vi "Interface.vi"(9 "EventsIn":T1, 10 "Events":T2) -> ()   [LabVIEW 2014, in "VIWindowProperties.lvlib" / "VIWindowProperties.lvclass"]
uses:
  VIWindowProperties.lvclass
  Framework/_Plugins/_LVCMPlugin/GCMPlugin_EventsOut.ctl
  Framework/_Plugins/_LVCMPlugin/GCMPlugin_EventsIn.ctl
  <vilib>/Utility/miscctls.llb/LVPointTypeDef.ctl
  Framework/_Plugins/GCMPlugin/GCMPlugin.lvclass
panel:
  in  "ToAP":bool
  in  "ToSP":bool
  in  "Tab Control":enum32{"Appearance", "Size and Position"}(tab)
  in  "Window has title bar":bool
  in  "Window behavior":enum32{"Default", "Floating", "Modal"}(radio)
  in  "Hide when LabVIEW in not active":bool
  in  "Window runs transparently":bool
  in  "Show menu bar":bool
  in  "Show vertical scroll bar":bool
  in  "Show horizontal scroll bar":bool
  in  "Show toolbar when running":bool
  in  "Show Abort button":bool
  in  "Show Run button":bool
  in  "Show Run Continuously":bool
  in  "Show front panel when called":bool
  in  "Close afterwards if originally closed":bool
  in  "Show front panel when loaded":bool
  in  "Transparently":u8 caption="Numeric Control"
  in  "Allow user to close window":bool
  in  "Allow user to resize window":bool
  in  "Allow user to minimalize window":bool
  in  "Allow default run time shortcut menus":bool
  in  "Highlight Enter boolean":bool
  in  "SP_SetCurrentSize":bool
  in  "SP_Height":i16 caption="Height"
  in  "SP_Width":i16 caption="Width"
  in  "SP_UseCurSize":bool caption="Use Current Panel Size"
  in  "SP_SetCurrentPos":bool
  in  "SP_Left":i16 caption="Left"
  in  "SP_Top":i16 caption="Top"
  in  "SP_UseCurPos":bool caption="Use Current Position"
  in  "SP_Scale":bool caption="Scale all objects on front panel as the window resizes"
  in  "SP_MinHeight":i16 caption="Height"
  in  "SP_MinWidth":i16 caption="Width"
  in  "SP_SetMinCurrent":bool
  in  "SP_proportions":bool caption="Maintain proportions of window for different monitor resolutions"
  in  "SP_Position":u16(ring) caption="Position" items=["Unchanged", "Centered", "Maximized", "Minimized", "Custom"]
  in  "SP_Monitor":u16(ring) caption="Monitor" items=["Primary", "1", "2", "3"]
  # "Window Size"
  # "Minimum Panel Size"
  # "Window Run-Time Position"
  # "Window Position"
  # "Panel Size"
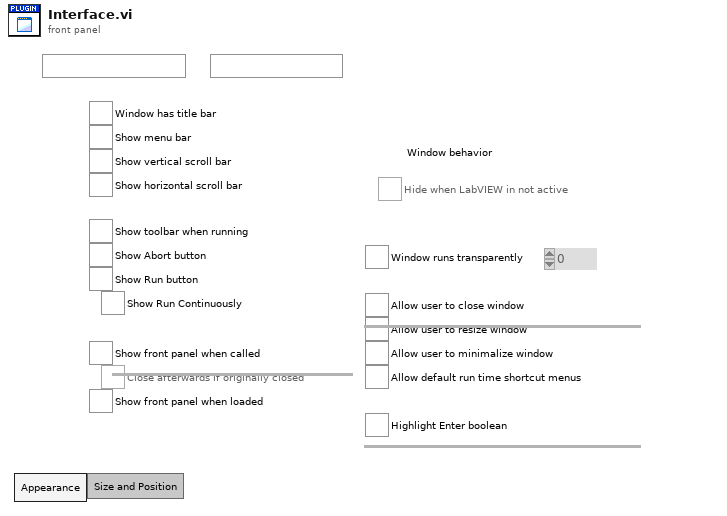
[diagram p1: front panel]
types:
  T1 = typedef "GCMPlugin.lvclass/GCMPlugin_EventsIn.ctl" = cluster{"Stop":refnum<user-event>, "ItemSelected":refnum<user-event>, "ItemDeselected":refnum<user-event>, "PluginActivated":refnum<user-event>, "PluginDeactivated":refnum<user-event>}
  T2 = typedef "GCMPlugin.lvclass/GCMPlugin_EventsOut.ctl" = cluster{"ItemEdited":refnum<user-event>}
  T3 = enum16{"No Scaling", "Scale All Objects", "Scale Single Object"}
  T4 = enum8{"Enabled", "Disabled", "Disabled and Grayed Out"}
  T5 = enum16{"Always On", "Always Off", "Off While Running"}
  T6 = typedef "LVPointTypeDef.ctl" = cluster{"Horizontal":i16, "Vertical":i16}
  T7 = enum32{"Invalid", "Default", "Floating", "Floating/Auto-Hide", "Modal"}
  T8 = enum32{"Unchanged", "Centered", "Maximized", "Minimized", "Custom"}
  T9 = typedef "LVRectTypeDef.ctl" = cluster{"Left":i16, "Top":i16, "Right":i16, "Bottom":i16}
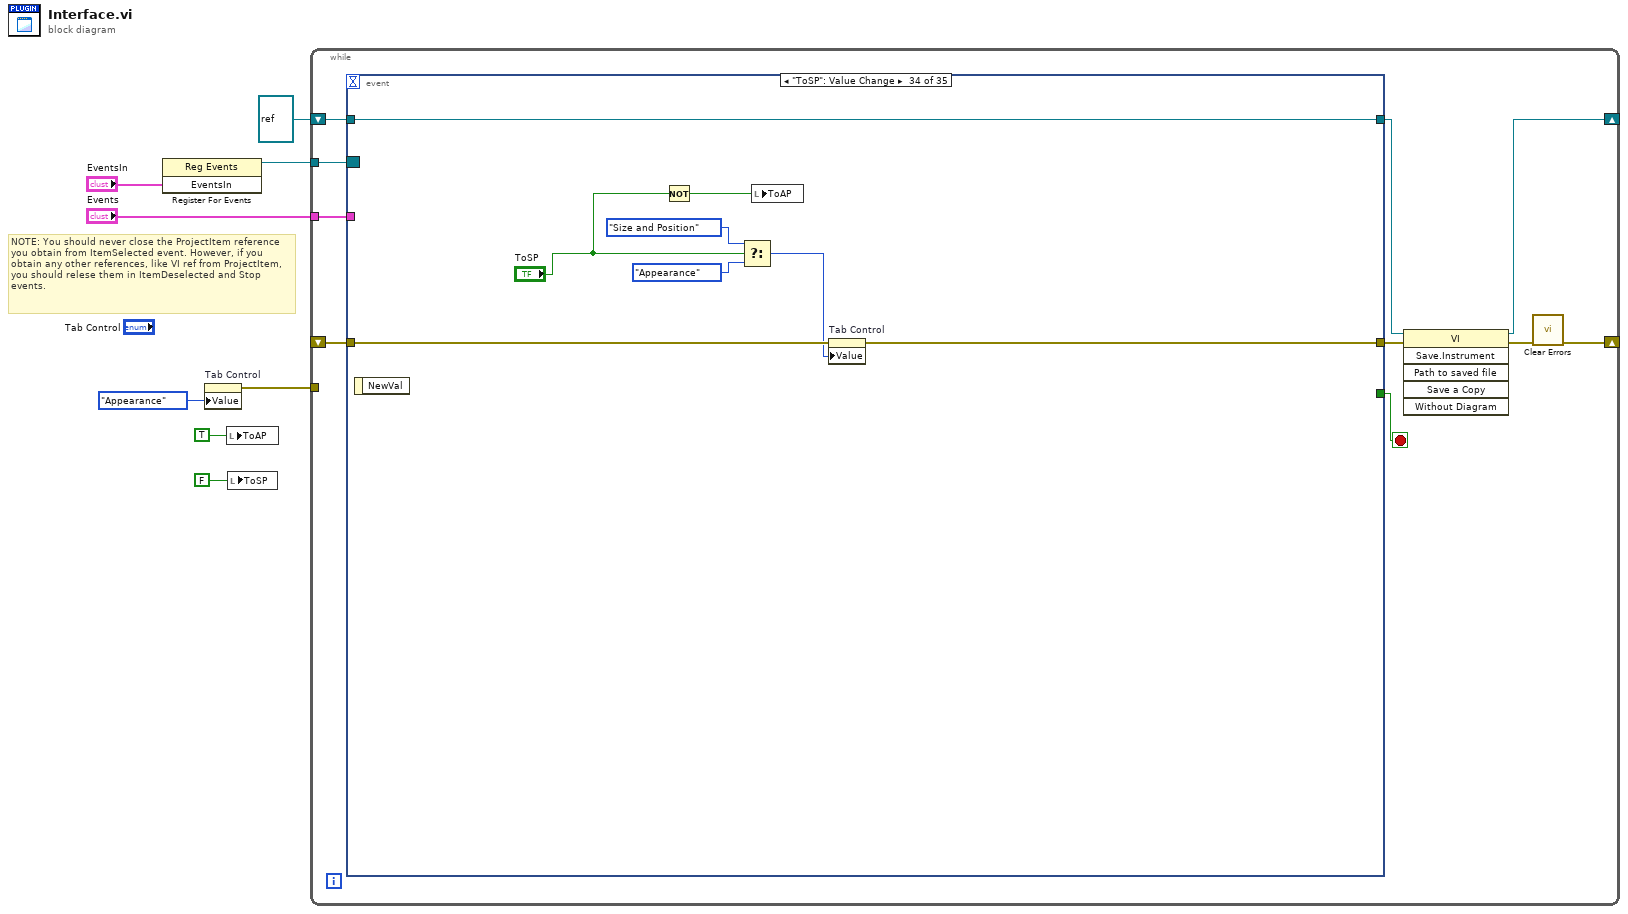
[diagram p0: block diagram]
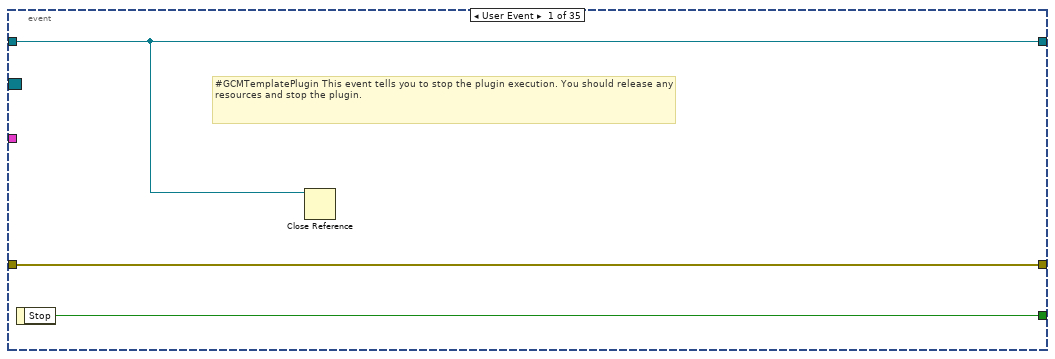
[diagram p2: hidden frame]
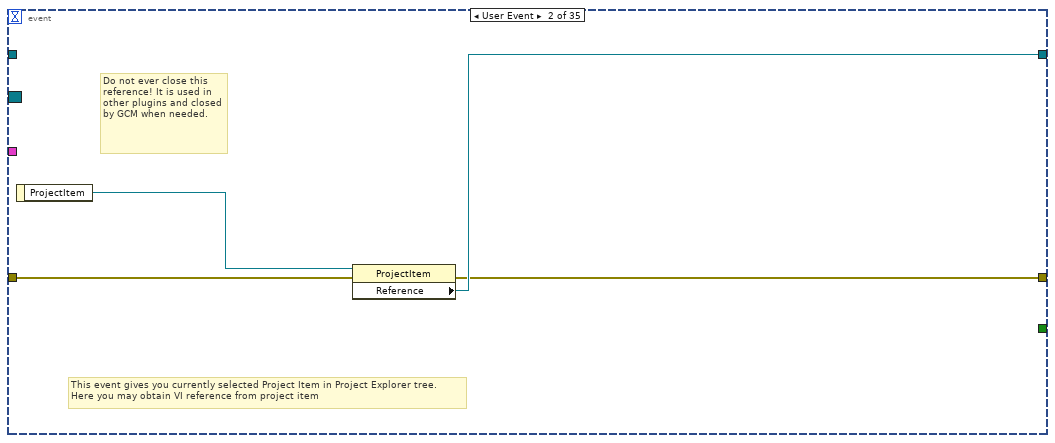
[diagram p3: hidden frame]
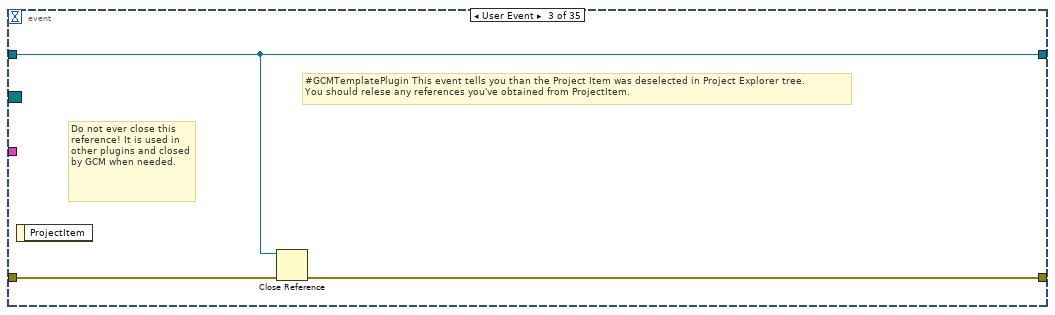
[diagram p4: hidden frame]
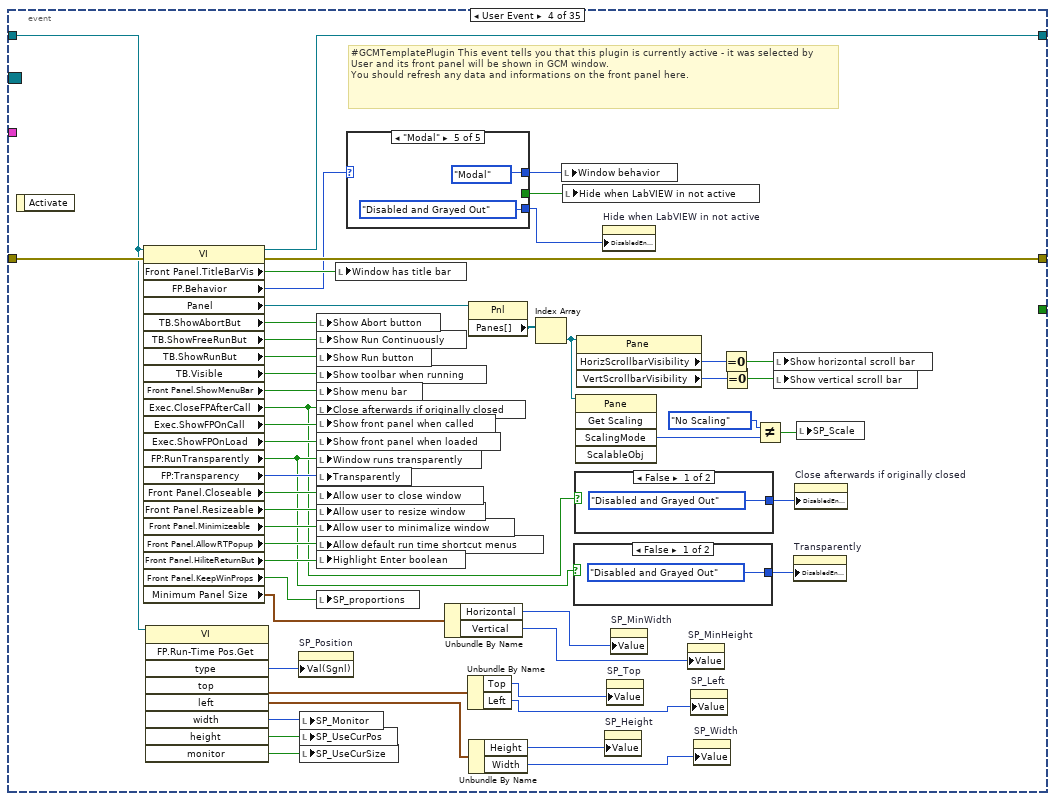
[diagram p5: hidden frame]
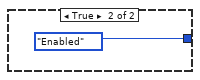
[diagram p6: hidden frame]
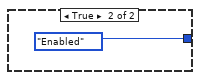
[diagram p7: hidden frame]
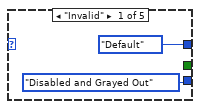
[diagram p8: hidden frame]
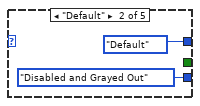
[diagram p9: hidden frame]
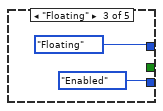
[diagram p10: hidden frame]
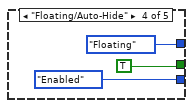
[diagram p11: hidden frame]
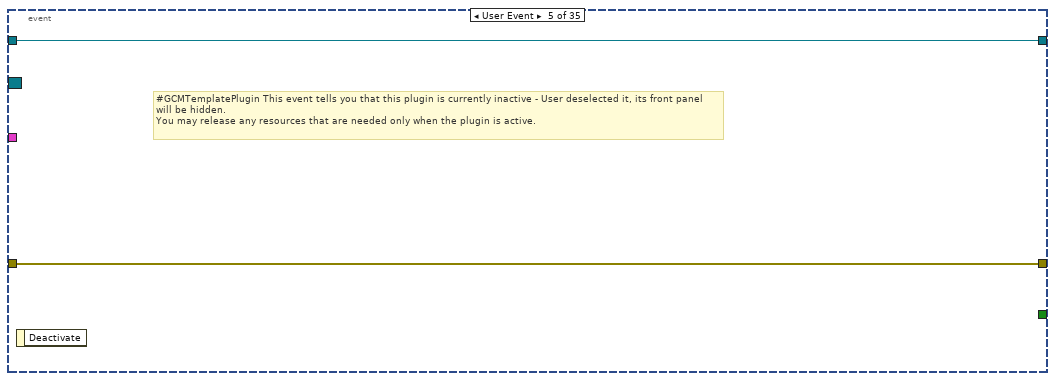
[diagram p12: hidden frame]
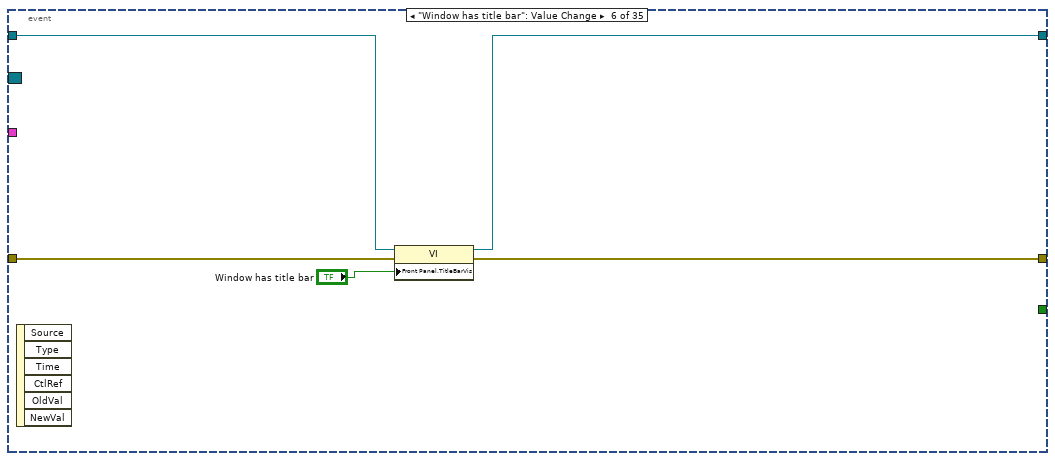
[diagram p13: hidden frame]
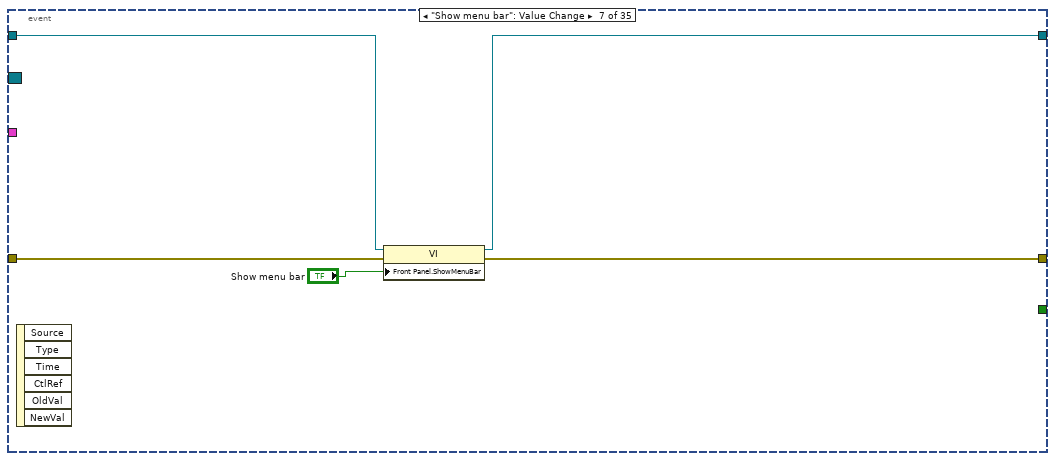
[diagram p14: hidden frame]
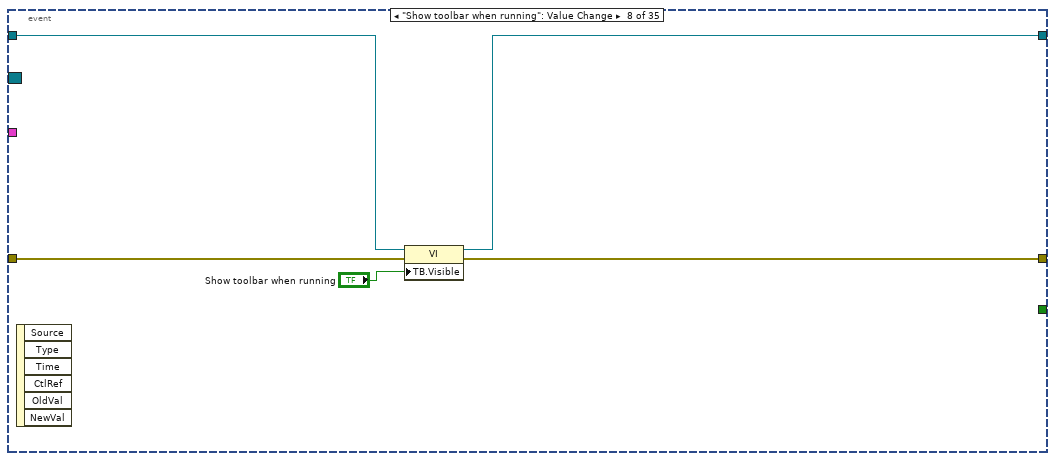
[diagram p15: hidden frame]
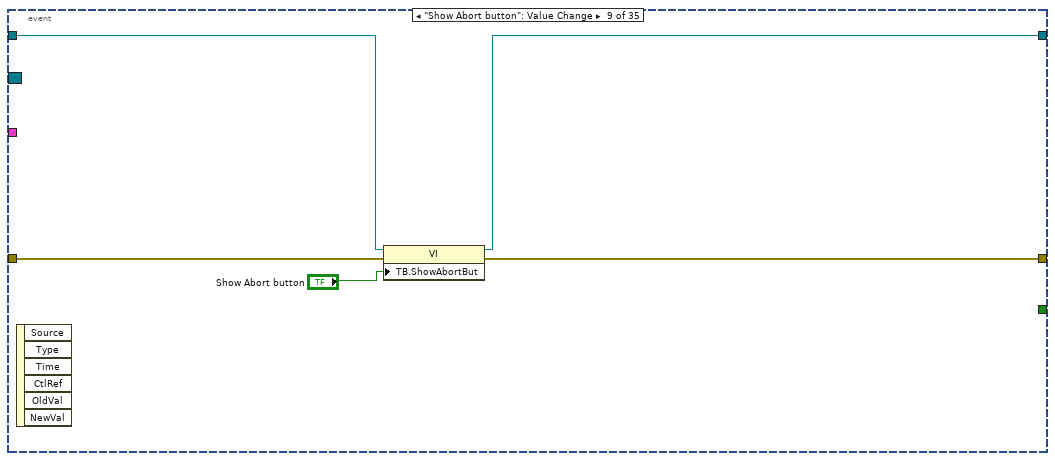
[diagram p16: hidden frame]
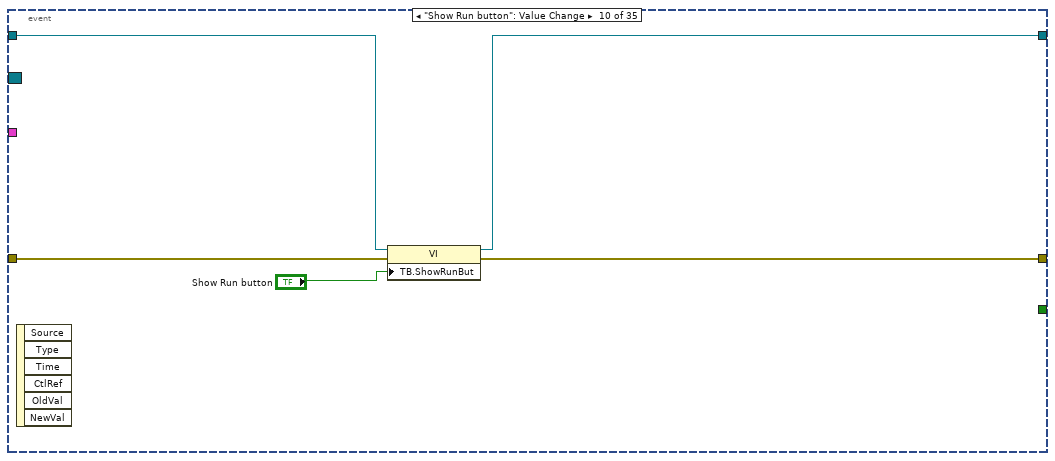
[diagram p17: hidden frame]
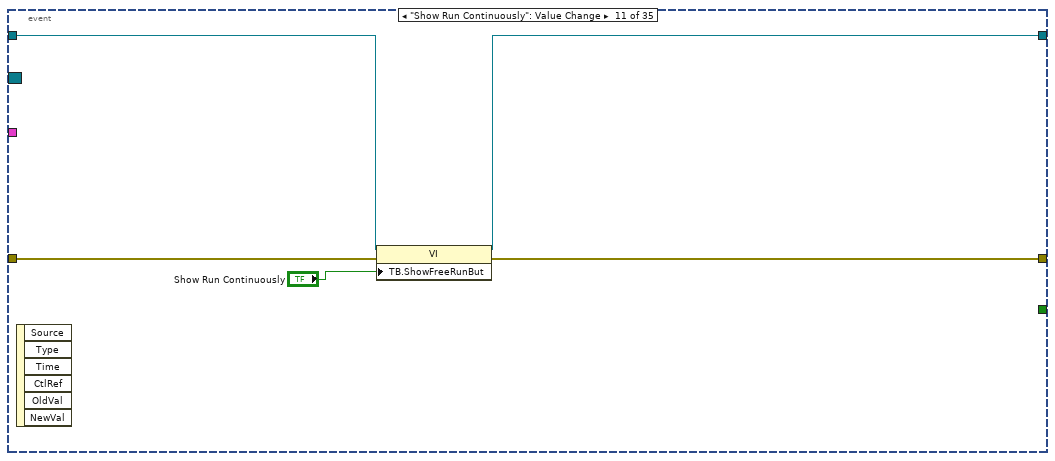
[diagram p18: hidden frame]
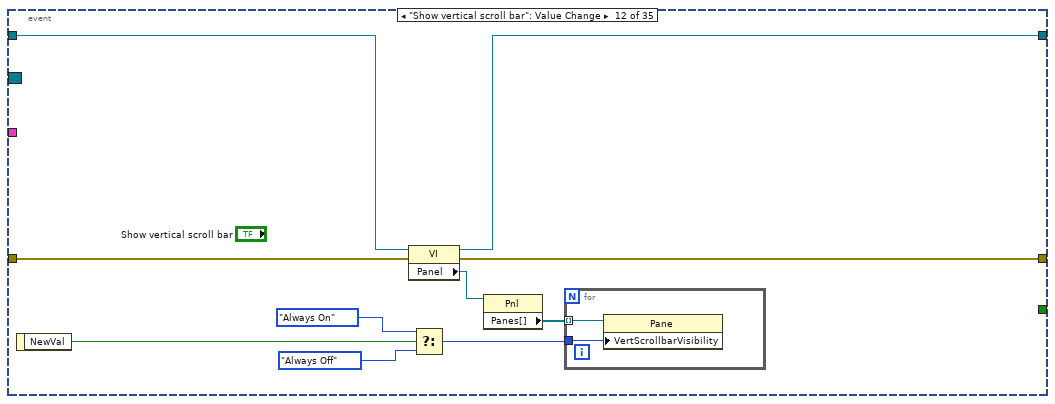
[diagram p19: hidden frame]
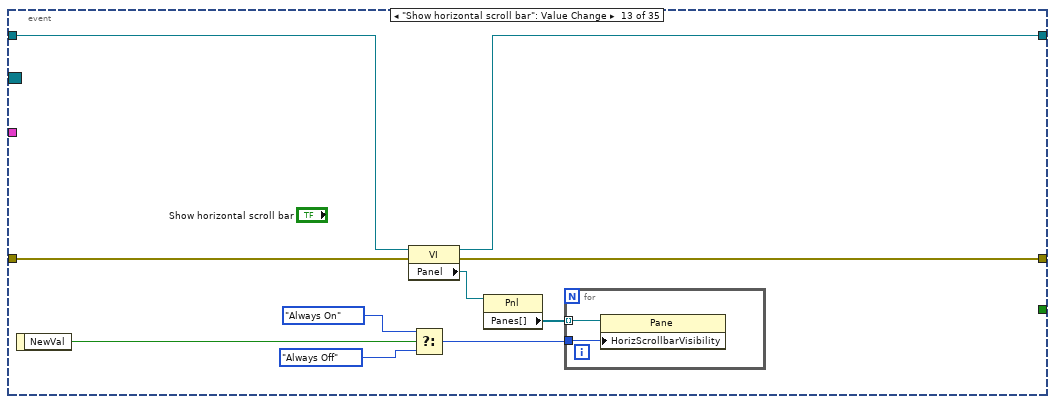
[diagram p20: hidden frame]
diagram:
  # "NOTE: You should never close the ProjectItem reference you obtain from ItemSelected event. However, if you obtain any other references, like VI ref from ProjectItem, you should relese them in ItemDeselected and Stop events."
  n1 = register-events("EventsIn") -> (reference out=w7:refnum<event-registration>)  [unwired: 2 in, 1 out]
  n2 = property on="Tab Control" class="TabCtl (strict)"("Value"=enum32{"Appearance", "Size and Position"}."Appearance" ("Tab Control")) -> (error out=w3:errorcluster)  [unwired: 2 in, 1 out]
  n3 = local write "ToAP"(TRUE ("ToAP")) -> ()
  n4 = local write "ToSP"(FALSE ("ToAP")) -> ()
  n5 = while {
    tunnel: w7 -> [w18]
    tunnel: "Events" -> [w17]
    shift-right: [w9] -> _
    shift-left: refnum<vi> refnum ("Reference") -> [w15]
    shift-right: [w12] -> _
    shift-left: _ -> [w13]
    tunnel: w3 -> [_]
    stop <- w16 stop-if-true
    n6 = event shown="[33] \"ToSP\": Value Change" {
      selector: w18 -> [_ _ _ _ _ _ _ _ _ _ _ _ _ _ _ _ _ _ _ _ _ _ _ _ _ _ _ _ _ _ _ _ _ _ _]
      dyn-events: _ -> [_ _ _ _ _ _ _ _ _ _ _ _ _ _ _ _ _ _ _ _ _ _ _ _ _ _ _ _ _ _ _ _ _ _ _]
      timeout: _ -> [_ _ _ _ _ _ _ _ _ _ _ _ _ _ _ _ _ _ _ _ _ _ _ _ _ _ _ _ _ _ _ _ _ _ _]
      tunnel: w17 -> [_ _ _ _ _ _ _ _ _ _ _ _ _ _ _ _ _ _ _ _ _ _ _ _ _ _ _ _ _ _ _ _ _ _ _]
      tunnel: [w21 _ _ _ _ _ _ _ _ _ _ _ _ _ _ _ _ _ _ _ _ _ _ _ _ _ _ _ _ _ _ _ _ _ _] -> w16
      tunnel: [w19 w24 w28 w75 w95 w97 w102 w107 w112 w117 w122 w132 w144 w153 w160 w165 w172 w179 w184 w189 w194 w199 w204 w209 w217 w234 w350 w355 w376 w399 w406 w417 w423 w443 w451] -> w10
      tunnel: w15 -> [w19 _ w28 w39 w95 w98 w103 w108 w113 w118 w123 w133 w145 w154 w161 w166 w173 w180 w185 w190 w195 w200 w205 w210 w218 w235 w347 w354 w375 w398 w405 w408 w424 w443 w451]
      tunnel: [w20 w23 w26 w77 w94 w99 w104 w109 w114 w119 w124 w134 w146 w155 w162 w167 w174 w181 w186 w191 w196 w201 w206 w211 w219 w236 w351 w356 w377 w400 w407 w416 w425 w441 w449] -> w14
      tunnel: w13 -> [w20 w22 w27 w78 w94 w100 w105 w110 w115 w120 w125 w135 w147 w156 w163 w168 w175 w182 w187 w192 w197 w202 w207 w212 w220 w237 w346 w353 w374 w397 w404 w418 w426 w442 w450]
      event User Event {
        # "#GCMTemplatePlugin This event tells you to stop the plugin execution. You should release any resources and stop the plugin."
        n7 = event-data() -> ("Stop"=w21:bool)  [unwired: 1 in]
        n8 = Close Reference(reference=w19) -> ()  [unwired: 1 in, 1 out]
      }
      event User Event {
        # "Do not ever close this reference! It is used in other plugins and closed by GCM when needed."
        # "This event gives you currently selected Project Item in Project Explorer tree.\nHere you may obtain VI reference from project item"
        n9 = event-data() -> ("ProjectItem"=w25:refnum<vi>)  [unwired: 1 in]
        n10 = property class="ProjectItem"(reference=w25, error in=w22) -> (error out=w23:errorcluster, "Reference"=w24:refnum<vi>)  [unwired: 1 out]
      }
      event User Event {
        # "Do not ever close this reference! It is used in other plugins and closed by GCM when needed."
        # "#GCMTemplatePlugin This event tells you than the Project Item was deselected in Project Explorer tree.\nYou should relese any references you've obtained from ProjectItem."
        n11 = event-data() -> ()  [unwired: 1 in, 1 out]
        n12 = Close Reference(reference=w28, error in (no error)=w27) -> (error out=w26:errorcluster)
      }
      event User Event {
        # "#GCMTemplatePlugin This event tells you that this plugin is currently active - it was selected by User and its front panel will be shown in GCM window.\nYou should refresh any data and informations on the front panel here."
        n13 = event-data() -> ()  [unwired: 1 in, 1 out]
        n14 = property class="VI"(reference=w39, error in=w78) -> (reference out=w75:refnum<vi>, error out=w77:errorcluster, "Front Panel.TitleBarVis"=w76:bool, "FP.Behavior"=w54:T7, "Panel"=w60:refnum<vi>, "TB.ShowAbortBut"=w70:bool, "TB.ShowFreeRunBut"=w71:bool, "TB.ShowRunBut"=w72:bool, "TB.Visible"=w73:bool, "Front Panel.ShowMenuBar"=w69:bool, "Exec.CloseFPAfterCall"=w49:bool, "Exec.ShowFPOnCall"=w68:bool, "Exec.ShowFPOnLoad"=w67:bool, "FP:RunTransparently"=w51:bool, "FP:Transparency"=w66:u8, "Front Panel.Closeable"=w65:bool, "Front Panel.Resizeable"=w64:bool, "Front Panel.Minimizeable"=w63:bool, "Front Panel.AllowRTPopup"=w62:bool, "Front Panel.HiliteReturnBut"=w61:bool, "Front Panel.KeepWinProps"=w47:bool, "Minimum Panel Size"=w42:T6)
        n15 = invoke class="VI" method="FP.Run-Time Pos.Get"(reference=w39) -> ("type"=w35:T8, "top"=w34:cluster{"Top":i16, "Left":i16}, "left"=w31:cluster{"Height":i16, "Width":i16}, "width"=w38:i16, "height"=w37:bool, "monitor"=w36:bool)  [unwired: 8 in, 3 out]
        n16 = property on="SP_Position" class="Ring (strict)"("Val(Sgnl)"=w35) -> ()  [unwired: 2 in, 2 out]
        n17 = local write "SP_Monitor"(w38) -> ()
        n18 = local write "SP_UseCurPos"(w37) -> ()
        n19 = local write "SP_UseCurSize"(w36) -> ()
        n20 = local write "Show Abort button"(w70) -> ()
        n21 = local write "Show Run Continuously"(w71) -> ()
        n22 = local write "Show Run button"(w72) -> ()
        n23 = local write "Show toolbar when running"(w73) -> ()
        n24 = local write "Show menu bar"(w69) -> ()
        n25 = local write "Close afterwards if originally closed"(w49) -> ()
        n26 = local write "Show front panel when called"(w68) -> ()
        n27 = local write "Show front panel when loaded"(w67) -> ()
        n28 = local write "Window runs transparently"(w51) -> ()
        n29 = local write "Transparently"(w66) -> ()
        n30 = local write "Allow user to close window"(w65) -> ()
        n31 = local write "Allow user to resize window"(w64) -> ()
        n32 = local write "Allow user to minimalize window"(w63) -> ()
        n33 = local write "Allow default run time shortcut menus"(w62) -> ()
        n34 = local write "Highlight Enter boolean"(w61) -> ()
        n35 = local write "SP_proportions"(w47) -> ()
        n36 = local write "Window has title bar"(w76) -> ()
        n37 = case shown="\"Modal\"" w54 {
          tunnel: [enum32{"Default", "Floating", "Modal"}."Default" ("Window behavior") enum32{"Default", "Floating", "Modal"}."Default" ("Window behavior") enum32{"Default", "Floating", "Modal"}."Floating" ("Window behavior") enum32{"Default", "Floating", "Modal"}."Floating" ("Window behavior") enum32{"Default", "Floating", "Modal"}."Modal" ("Window behavior")] -> w48
          tunnel: [_ _ _ TRUE _] -> w74
          tunnel: [T4."Disabled and Grayed Out" ("Disabled") T4."Disabled and Grayed Out" ("Disabled") T4."Enabled" ("Disabled") T4."Enabled" ("Disabled") T4."Disabled and Grayed Out" ("Disabled")] -> w53
          frame "Invalid" {
          }
          frame "Default" {
          }
          frame "Floating" {
          }
          frame "Floating/Auto-Hide" {
          }
          frame "Modal" {
          }
        }
        n38 = Unbundle By Name(w42) -> ("Horizontal"=w41:i16, "Vertical"=w40:i16)
        n39 = Unbundle By Name(w34) -> ("Top"=w33:i16, "Left"=w32:i16)
        n40 = property class="Pnl"(reference=w60) -> ("Panes[]"=w59:refnum<vi>[])  [unwired: 1 in, 2 out]
        n41 = Unbundle By Name(w31) -> ("Height"=w30:i16, "Width"=w29:i16)
        n42 = Index Array(array=w59) -> (element=w46:refnum<vi>)  [unwired: 1 in]
        n43 = local write "Window behavior"(w48) -> ()
        n44 = local write "Hide when LabVIEW in not active"(w74) -> ()
        n45 = case shown="False" w51 {
          tunnel: [T4."Disabled and Grayed Out" ("Disabled") T4."Enabled" ("Disabled")] -> w52
          frame False {
          }
          frame True {
          }
        }
        n46 = case shown="False" w49 {
          tunnel: [T4."Disabled and Grayed Out" ("Disabled") T4."Enabled" ("Disabled")] -> w50
          frame False {
          }
          frame True {
          }
        }
        n47 = invoke class="Pane" method="Get Scaling"(reference=w46) -> ("ScalingMode"=w45:T3)  [unwired: 4 in, 4 out]
        n48 = property class="Pane"(reference=w46) -> ("HorizScrollbarVisibility"=w58:T5, "VertScrollbarVisibility"=w57:T5)  [unwired: 1 in, 2 out]
        n49 = property on="Hide when LabVIEW in not active" class="Bool (strict)"("DisabledEnum"=w53) -> ()  [unwired: 2 in, 2 out]
        n50 = property on="SP_Height" class="DigNum (strict)"("Value"=w30) -> ()  [unwired: 2 in, 2 out]
        n51 = property on="SP_Top" class="DigNum (strict)"("Value"=w33) -> ()  [unwired: 2 in, 2 out]
        n52 = property on="SP_MinWidth" class="DigNum (strict)"("Value"=w41) -> ()  [unwired: 2 in, 2 out]
        n53 = property on="SP_MinHeight" class="DigNum (strict)"("Value"=w40) -> ()  [unwired: 2 in, 2 out]
        n54 = property on="SP_Left" class="DigNum (strict)"("Value"=w32) -> ()  [unwired: 2 in, 2 out]
        n55 = property on="SP_Width" class="DigNum (strict)"("Value"=w29) -> ()  [unwired: 2 in, 2 out]
        n56 = Equal To 0?(x=w58) -> (x = 0?=w56:bool)
        n57 = Equal To 0?(x=w57) -> (x = 0?=w55:bool)
        n58 = Not Equal?(x=T3."No Scaling", y=w45) -> (x != y?=w43:bool)
        n59 = local write "Show horizontal scroll bar"(w56) -> ()
        n60 = local write "Show vertical scroll bar"(w55) -> ()
        n61 = property on="Transparently" class="DigNum (strict)"("DisabledEnum"=w52) -> ()  [unwired: 2 in, 2 out]
        n62 = property on="Close afterwards if originally closed" class="Bool (strict)"("DisabledEnum"=w50) -> ()  [unwired: 2 in, 2 out]
        n63 = local write "SP_Scale"(w43) -> ()
      }
      event User Event {
        # "#GCMTemplatePlugin This event tells you that this plugin is currently inactive - User deselected it, its front panel will be hidden.\nYou may release any resources that are needed only when the plugin is active."
        n64 = event-data() -> ()  [unwired: 1 in, 1 out]
      }
      event "Window has title bar": Value Change {
        n65 = event-data() -> ()  [unwired: 1 in, 6 out]
        n66 = property class="VI"(reference=w98, error in=w100, "Front Panel.TitleBarVis"="Window has title bar") -> (reference out=w97:refnum<vi>, error out=w99:errorcluster)
      }
      event "Show menu bar": Value Change {
        n67 = event-data() -> ()  [unwired: 1 in, 6 out]
        n68 = property class="VI"(reference=w103, error in=w105, "Front Panel.ShowMenuBar"="Show menu bar") -> (reference out=w102:refnum<vi>, error out=w104:errorcluster)
      }
      event "Show toolbar when running": Value Change {
        n69 = event-data() -> ()  [unwired: 1 in, 6 out]
        n70 = property class="VI"(reference=w108, error in=w110, "TB.Visible"="Show toolbar when running") -> (reference out=w107:refnum<vi>, error out=w109:errorcluster)
      }
      event "Show Abort button": Value Change {
        n71 = event-data() -> ()  [unwired: 1 in, 6 out]
        n72 = property class="VI"(reference=w113, error in=w115, "TB.ShowAbortBut"="Show Abort button") -> (reference out=w112:refnum<vi>, error out=w114:errorcluster)
      }
      event "Show Run button": Value Change {
        n73 = event-data() -> ()  [unwired: 1 in, 6 out]
        n74 = property class="VI"(reference=w118, error in=w120, "TB.ShowRunBut"="Show Run button") -> (reference out=w117:refnum<vi>, error out=w119:errorcluster)
      }
      event "Show Run Continuously": Value Change {
        n75 = event-data() -> ()  [unwired: 1 in, 6 out]
        n76 = property class="VI"(reference=w123, error in=w125, "TB.ShowFreeRunBut"="Show Run Continuously") -> (reference out=w122:refnum<vi>, error out=w124:errorcluster)
      }
      event "Show vertical scroll bar": Value Change {
        n77 = event-data() -> ("NewVal"=w129:bool)  [unwired: 1 in]
        n78 = property class="VI"(reference=w133, error in=w135) -> (reference out=w132:refnum<vi>, error out=w134:errorcluster, "Panel"=w131:refnum<vi>)
        n79 = Select(t=T5."Always On" ("Vertical Scrollbar Visibility"), s=w129, f=T5."Always Off" ("Vertical Scrollbar Visibility")) -> (s? t:f=w126:T5)
        n80 = property class="Pnl"(reference=w131) -> ("Panes[]"=w130:refnum<vi>[])  [unwired: 1 in, 2 out]
        n81 = for {
          tunnel: w130 -> [w137] mode=indexing
          tunnel: w126 -> [w136]
          n82 = property class="Pane"(reference=w137, "VertScrollbarVisibility"=w136) -> ()  [unwired: 1 in, 2 out]
        }
      }
      event "Show horizontal scroll bar": Value Change {
        n83 = event-data() -> ("NewVal"=w141:bool)  [unwired: 1 in]
        n84 = property class="VI"(reference=w145, error in=w147) -> (reference out=w144:refnum<vi>, error out=w146:errorcluster, "Panel"=w143:refnum<vi>)
        n85 = Select(t=T5."Always On" ("Vertical Scrollbar Visibility"), s=w141, f=T5."Always Off" ("Vertical Scrollbar Visibility")) -> (s? t:f=w138:T5)
        n86 = property class="Pnl"(reference=w143) -> ("Panes[]"=w142:refnum<vi>[])  [unwired: 1 in, 2 out]
        n87 = for {
          tunnel: w142 -> [w149] mode=indexing
          tunnel: w138 -> [w148]
          n88 = property class="Pane"(reference=w149, "HorizScrollbarVisibility"=w148) -> ()  [unwired: 1 in, 2 out]
        }
      }
      event "Show front panel when called": Value Change {
        n89 = event-data() -> ("NewVal"=w150:bool)  [unwired: 1 in, 5 out]
        n90 = case shown="False" w150 {
          tunnel: [T4."Disabled and Grayed Out" ("Disabled") T4."Enabled" ("Disabled")] -> w151
          frame False {
          }
          frame True {
          }
        }
        n91 = property on="Close afterwards if originally closed" class="Bool (strict)"("DisabledEnum"=w151) -> ()  [unwired: 2 in, 2 out]
        n92 = property class="VI"(reference=w154, error in=w156, "Exec.ShowFPOnCall"="Show front panel when called") -> (reference out=w153:refnum<vi>, error out=w155:errorcluster)
      }
      event "Close afterwards if originally closed": Value Change {
        n93 = event-data() -> ()  [unwired: 1 in, 6 out]
        n94 = property class="VI"(reference=w161, error in=w163, "Exec.CloseFPAfterCall"="Close afterwards if originally closed") -> (reference out=w160:refnum<vi>, error out=w162:errorcluster)
      }
      event "Show front panel when loaded": Value Change {
        n95 = event-data() -> ()  [unwired: 1 in, 6 out]
        n96 = property class="VI"(reference=w166, error in=w168, "Exec.ShowFPOnLoad"="Show front panel when loaded") -> (reference out=w165:refnum<vi>, error out=w167:errorcluster)
      }
      event "Window runs transparently": Value Change {
        n97 = event-data() -> ("NewVal"=w170:bool)  [unwired: 1 in, 5 out]
        n98 = case shown="False" w170 {
          tunnel: [T4."Disabled and Grayed Out" ("Disabled") T4."Enabled" ("Disabled")] -> w169
          frame False {
          }
          frame True {
          }
        }
        n99 = property class="VI"(reference=w173, error in=w175, "FP:RunTransparently"="Window runs transparently") -> (reference out=w172:refnum<vi>, error out=w174:errorcluster)
        n100 = property on="Transparently" class="DigNum (strict)"("DisabledEnum"=w169) -> ()  [unwired: 2 in, 2 out]
      }
      event "Allow user to close window": Value Change {
        n101 = event-data() -> ()  [unwired: 1 in, 6 out]
        n102 = property class="VI"(reference=w180, error in=w182, "Front Panel.Closeable"="Allow user to close window") -> (reference out=w179:refnum<vi>, error out=w181:errorcluster)
      }
      event "Allow user to resize window": Value Change {
        n103 = event-data() -> ()  [unwired: 1 in, 6 out]
        n104 = property class="VI"(reference=w185, error in=w187, "Front Panel.Resizeable"="Allow user to resize window") -> (reference out=w184:refnum<vi>, error out=w186:errorcluster)
      }
      event "Allow user to minimalize window": Value Change {
        n105 = event-data() -> ()  [unwired: 1 in, 6 out]
        n106 = property class="VI"(reference=w190, error in=w192, "Front Panel.Minimizeable"="Allow user to minimalize window") -> (reference out=w189:refnum<vi>, error out=w191:errorcluster)
      }
      event "Allow default run time shortcut menus": Value Change {
        n107 = event-data() -> ()  [unwired: 1 in, 6 out]
        n108 = property class="VI"(reference=w195, error in=w197, "Front Panel.AllowRTPopup"="Allow default run time shortcut menus") -> (reference out=w194:refnum<vi>, error out=w196:errorcluster)
      }
      event "Highlight Enter boolean": Value Change {
        n109 = event-data() -> ()  [unwired: 1 in, 6 out]
        n110 = property class="VI"(reference=w200, error in=w202, "Front Panel.HiliteReturnBut"="Highlight Enter boolean") -> (reference out=w199:refnum<vi>, error out=w201:errorcluster)
      }
      event "SP_proportions": Value Change {
        n111 = event-data() -> ()  [unwired: 1 in, 6 out]
        n112 = property class="VI"(reference=w205, error in=w207, "Front Panel.KeepWinProps"="SP_proportions") -> (reference out=w204:refnum<vi>, error out=w206:errorcluster)
      }
      event "Transparently": Value Change {
        n113 = event-data() -> ()  [unwired: 1 in, 6 out]
        n114 = property class="VI"(reference=w210, error in=w212, "FP:Transparency"="Transparently") -> (reference out=w209:refnum<vi>, error out=w211:errorcluster)
      }
      event "SP_MinWidth", "SP_MinHeight": Value Change {
        n115 = event-data() -> ()  [unwired: 1 in, 6 out]
        n116 = Bundle By Name(cluster=T6 {"Horizontal"=0, "Vertical"=0} ("Front Panel Window:Minimum Size"), "Horizontal"="SP_MinWidth", "Vertical"="SP_MinHeight") -> (w213:T6)
        n117 = property class="VI"(reference=w218, error in=w220, "Minimum Panel Size"=w213) -> (reference out=w217:refnum<vi>, error out=w219:errorcluster)
      }
      event "SP_Position", "SP_Monitor", "SP_Top", "SP_Left", "SP_Width", "SP_Height": Value Change {
        n118 = event-data() -> ()  [unwired: 1 in, 6 out]
        n119 = property on="SP_UseCurSize" class="Bool (strict)"() -> ("Value"=w222:bool)  [unwired: 2 in, 2 out]
        n120 = property on="SP_UseCurPos" class="Bool (strict)"() -> ("Value"=w221:bool)  [unwired: 2 in, 2 out]
        n121 = case shown="3" "SP_Position" {
          tunnel: w237 -> [w242 w266 w280 w287 w319]
          tunnel: [w239 w263 w278 w285 w318] -> w236
          tunnel: w235 -> [w241 w265 w281 w288 w316]
          tunnel: [w240 w264 w279 w286 w317] -> w234
          tunnel: w221 -> [_ _ _ _ w296]
          tunnel: "SP_Top" -> [_ _ _ _ w312]
          tunnel: "SP_Left" -> [_ _ _ _ w311]
          tunnel: w222 -> [_ w246 _ _ w293]
          tunnel: "SP_Width" -> [_ w245 _ _ w301]
          tunnel: "SP_Height" -> [_ w244 _ _ w300]
          tunnel: "SP_Monitor" -> [_ w256 w277 w284 _]
          tunnel: [w238 w260 T4."Enabled" ("Disabled") T4."Enabled" ("Disabled") T4."Disabled and Grayed Out" ("Disabled")] -> w227
          tunnel: [w238 w261 w275 w282 w297] -> w225
          tunnel: [w238 w261 w275 w282 w292] -> w224
          tunnel: [w238 w260 w275 w282 w297] -> w226
          tunnel: [w238 w262 w275 w282 w291] -> w223
          frame 0, Default {
            w238 = T4."Disabled and Grayed Out" ("Disabled")
            # "Unchanged"
            n122 = invoke class="VI" method="FP.Run-Time Pos.Unchanged"(reference=w241, error in=w242) -> (reference out=w240:refnum<vi>, error out=w239:errorcluster)  [unwired: 1 in, 1 out]
          }
          frame 1 {
            w261 = T4."Disabled and Grayed Out" ("Disabled")
            w260 = T4."Enabled" ("Disabled")
            # "Centred"
            n123 = property class="VI"(reference=w265, error in=w266) -> (reference out=w258:refnum<vi>, error out=w257:errorcluster, "Front Panel.PanelBounds"=w247:T9)
            n124 = Unbundle By Name(w247) -> ("Left"=w255:i16, "Right"=w254:i16, "Top"=w253:i16, "Bottom"=w252:i16)
            n125 = Subtract(x=w255, y=w254) -> (x-y=w251:i16)
            n126 = Subtract(x=w253, y=w252) -> (x-y=w250:i16)
            n127 = Absolute Value(x=w251) -> (abs(x)=w249:i16)
            n128 = Absolute Value(x=w250) -> (abs(x)=w248:i16)
            n129 = case shown="False" w246 {
              tunnel: w249 -> [w269 _]
              tunnel: w248 -> [w268 _]
              tunnel: w245 -> [_ w273]
              tunnel: w244 -> [_ w272]
              tunnel: [w267 w271] -> w243
              frame True {
                n130 = Bundle By Name(cluster=cluster{"Height":i16, "Width":i16} {"Height"=0, "Width"=0} ("Size"), "Width"=w269, "Height"=w268) -> (w267:cluster{"Height":i16, "Width":i16})
              }
              frame False {
                n131 = Bundle By Name(cluster=cluster{"Height":i16, "Width":i16} {"Height"=0, "Width"=0} ("Size"), "Width"=w273, "Height"=w272) -> (w271:cluster{"Height":i16, "Width":i16})
              }
            }
            n132 = Not(x=w246) -> (.not. x?=w259:bool)
            n133 = invoke class="VI" method="FP.Run-Time Position.Centered"(reference=w258, error in=w257, "Monitor"=w256, "Monitor"=w243) -> (reference out=w264:refnum<vi>, error out=w263:errorcluster)  [unwired: 1 in, 3 out]
            n134 = Select(t=w260, s=w259, f=w261) -> (s? t:f=w262:T4)
          }
          frame 2 {
            w275 = T4."Disabled and Grayed Out" ("Disabled")
            # "Maximalized"
            n135 = invoke class="VI" method="FP.Run-Time Position.Maximized"(reference=w281, error in=w280, "Monitor"=w277) -> (reference out=w279:refnum<vi>, error out=w278:errorcluster)  [unwired: 1 in, 2 out]
          }
          frame 3 {
            w282 = T4."Disabled and Grayed Out" ("Disabled")
            # "Minimalized"
            n136 = invoke class="VI" method="FP.Run-Time Position.Minimized"(reference=w288, error in=w287, "Monitor"=w284) -> (reference out=w286:refnum<vi>, error out=w285:errorcluster)  [unwired: 1 in, 2 out]
          }
          frame 4 {
            w294 = T4."Disabled and Grayed Out" ("Disabled")
            w295 = T4."Enabled" ("Disabled")
            w297 = T4."Enabled" ("Disabled")
            # "Custom"
            n137 = property class="VI"(reference=w316) -> ("Front Panel.PanelBounds"=w304:T9)  [unwired: 1 in, 2 out]
            n138 = Unbundle By Name(w304) -> ("Left"=w310:i16, "Right"=w309:i16, "Top"=w308:i16, "Bottom"=w307:i16)
            n139 = Subtract(x=w310, y=w309) -> (x-y=w306:i16)
            n140 = Subtract(x=w308, y=w307) -> (x-y=w305:i16)
            n141 = Unbundle By Name(w304) -> ("Top"=w315:i16, "Left"=w314:i16)
            n142 = Not(x=w293) -> (.not. x?=w289:bool)
            n143 = Not(x=w296) -> (.not. x?=w290:bool)
            n144 = Absolute Value(x=w306) -> (abs(x)=w303:i16)
            n145 = Absolute Value(x=w305) -> (abs(x)=w302:i16)
            n146 = case shown="False" w296 {
              tunnel: w315 -> [w330 _]
              tunnel: w314 -> [w329 _]
              tunnel: [w328 w334] -> w313
              tunnel: w312 -> [_ w333]
              tunnel: w311 -> [_ w332]
              frame True {
                n147 = Bundle By Name(cluster=cluster{"Top":i16, "Left":i16} {"Top"=0, "Left"=0} ("Position"), "Top"=w330, "Left"=w329) -> (w328:cluster{"Top":i16, "Left":i16})
              }
              frame False {
                n148 = Bundle By Name(cluster=cluster{"Top":i16, "Left":i16} {"Top"=0, "Left"=0} ("Position"), "Top"=w333, "Left"=w332) -> (w334:cluster{"Top":i16, "Left":i16})
              }
            }
            n149 = case shown="True" w293 {
              tunnel: w303 -> [w322 _]
              tunnel: w302 -> [w321 _]
              tunnel: w301 -> [_ w326]
              tunnel: w300 -> [_ w325]
              tunnel: [w320 w324] -> w299
              frame True {
                n150 = Bundle By Name(cluster=cluster{"Height":i16, "Width":i16} {"Height"=0, "Width"=0} ("Size"), "Width"=w322, "Height"=w321) -> (w320:cluster{"Height":i16, "Width":i16})
              }
              frame False {
                n151 = Bundle By Name(cluster=cluster{"Height":i16, "Width":i16} {"Height"=0, "Width"=0} ("Size"), "Width"=w326, "Height"=w325) -> (w324:cluster{"Height":i16, "Width":i16})
              }
            }
            n152 = invoke class="VI" method="FP.Run-Time Position.Custom"(reference=w316, error in=w319, "Size"=w313, "Position"=w299) -> (reference out=w317:refnum<vi>, error out=w318:errorcluster)  [unwired: 1 in, 3 out]
            n153 = Select(t=w295, s=w290, f=w294) -> (s? t:f=w292:T4)
            n154 = Select(t=w295, s=w289, f=w294) -> (s? t:f=w291:T4)
          }
        }
        n155 = property on="SP_Monitor" class="Ring (strict)"("DisabledEnum"=w227) -> ()  [unwired: 2 in, 2 out]
        n156 = property on="SP_UseCurPos" class="Bool (strict)"("DisabledEnum"=w225) -> ()  [unwired: 2 in, 2 out]
        n157 = property on="SP_Left" class="DigNum (strict)"("DisabledEnum"=w224) -> ()  [unwired: 2 in, 2 out]
        n158 = property on="SP_Top" class="DigNum (strict)"("DisabledEnum"=w224) -> ()  [unwired: 2 in, 2 out]
        n159 = property on="SP_UseCurSize" class="Bool (strict)"("DisabledEnum"=w226) -> ()  [unwired: 2 in, 2 out]
        n160 = property on="SP_Width" class="DigNum (strict)"("DisabledEnum"=w223) -> ()  [unwired: 2 in, 2 out]
        n161 = property on="SP_Height" class="DigNum (strict)"("DisabledEnum"=w223) -> ()  [unwired: 2 in, 2 out]
        n162 = property on="SP_SetCurrentSize" class="Bool"("DisabledEnum"=w223) -> ()  [unwired: 2 in, 2 out]
        n163 = property on="SP_SetCurrentPos" class="Bool"("DisabledEnum"=w224) -> ()  [unwired: 2 in, 2 out]
      }
      event "SP_SetMinCurrent": Value Change {
        n164 = event-data() -> ()  [unwired: 1 in, 6 out]
        n165 = property class="VI"(reference=w347, error in=w346) -> (reference out=w345:refnum<vi>, "Front Panel.PanelBounds"=w344:T9)  [unwired: 1 out]
        n166 = Unbundle By Name(w344) -> ("Left"=w343:i16, "Right"=w342:i16, "Top"=w341:i16, "Bottom"=w340:i16)
        n167 = Subtract(x=w343, y=w342) -> (x-y=w339:i16)
        n168 = Subtract(x=w341, y=w340) -> (x-y=w338:i16)
        n169 = Absolute Value(x=w339) -> (abs(x)=w337:i16)
        n170 = Absolute Value(x=w338) -> (abs(x)=w336:i16)
        n171 = Bundle By Name(cluster=T6 {"Horizontal"=0, "Vertical"=0} ("Front Panel Window:Minimum Size"), "Horizontal"=w337, "Vertical"=w336) -> (w348:T6)
        n172 = property on="SP_MinWidth" class="DigNum (strict)"("Value"=w337) -> ()  [unwired: 2 in, 2 out]
        n173 = property on="SP_MinHeight" class="DigNum (strict)"("Value"=w336) -> ()  [unwired: 2 in, 2 out]
        n174 = property class="VI"(reference=w345, "Minimum Panel Size"=w348) -> (reference out=w350:refnum<vi>, error out=w351:errorcluster)  [unwired: 1 in]
      }
      event "SP_UseCurSize": Value Change {
        n175 = event-data() -> ("NewVal"=w352:bool)  [unwired: 1 in]
        n176 = case shown="False" w352 {
          tunnel: [w358 w372] -> w356
          tunnel: [w359 w371] -> w355
          tunnel: w354 -> [w359 w370]
          tunnel: w353 -> [w358 w369]
          frame False {
            n177 = property on="SP_Position" class="Ring (strict)"() -> ("Value"=w357:u16)  [unwired: 2 in, 2 out]
            n178 = property on="SP_Position" class="Ring (strict)"("Val(Sgnl)"=w357) -> ()  [unwired: 2 in, 2 out]
          }
          frame True {
            n179 = property class="VI"(reference=w370, error in=w369) -> (reference out=w371:refnum<vi>, error out=w372:errorcluster, "Front Panel.PanelBounds"=w368:T9)
            n180 = Unbundle By Name(w368) -> ("Left"=w367:i16, "Right"=w366:i16, "Top"=w365:i16, "Bottom"=w364:i16)
            n181 = Subtract(x=w367, y=w366) -> (x-y=w363:i16)
            n182 = Subtract(x=w365, y=w364) -> (x-y=w362:i16)
            n183 = Absolute Value(x=w363) -> (abs(x)=w360:i16)
            n184 = Absolute Value(x=w362) -> (abs(x)=w361:i16)
            n185 = property on="SP_Width" class="DigNum (strict)"("Val(Sgnl)"=w360) -> ()  [unwired: 2 in, 2 out]
            n186 = property on="SP_Height" class="DigNum (strict)"("Value"=w361) -> ()  [unwired: 2 in, 2 out]
          }
        }
      }
      event "SP_UseCurPos": Value Change {
        n187 = event-data() -> ("NewVal"=w373:bool)  [unwired: 1 in]
        n188 = case shown="True" w373 {
          tunnel: [w379 w387] -> w377
          tunnel: [w380 w386] -> w376
          tunnel: w375 -> [w380 w385]
          tunnel: w374 -> [w379 w384]
          frame False {
            n189 = property on="SP_Position" class="Ring (strict)"() -> ("Value"=w378:u16)  [unwired: 2 in, 2 out]
            n190 = property on="SP_Position" class="Ring (strict)"("Val(Sgnl)"=w378) -> ()  [unwired: 2 in, 2 out]
          }
          frame True {
            n191 = property class="VI"(reference=w385, error in=w384) -> (reference out=w386:refnum<vi>, error out=w387:errorcluster, "Front Panel.PanelBounds"=w383:T9)
            n192 = Unbundle By Name(w383) -> ("Left"=w382:i16, "Top"=w381:i16)
            n193 = property on="SP_Left" class="DigNum (strict)"("Val(Sgnl)"=w382) -> ()  [unwired: 2 in, 2 out]
            n194 = property on="SP_Top" class="DigNum (strict)"("Value"=w381) -> ()  [unwired: 2 in, 2 out]
          }
        }
      }
      event "SP_SetCurrentSize": Value Change {
        n195 = event-data() -> ()  [unwired: 1 in, 1 out]
        n196 = property class="VI"(reference=w398, error in=w397) -> (reference out=w399:refnum<vi>, error out=w400:errorcluster, "Front Panel.PanelBounds"=w396:T9)
        n197 = Unbundle By Name(w396) -> ("Left"=w395:i16, "Right"=w394:i16, "Top"=w393:i16, "Bottom"=w392:i16)
        n198 = Subtract(x=w395, y=w394) -> (x-y=w391:i16)
        n199 = Subtract(x=w393, y=w392) -> (x-y=w390:i16)
        n200 = Absolute Value(x=w391) -> (abs(x)=w388:i16)
        n201 = Absolute Value(x=w390) -> (abs(x)=w389:i16)
        n202 = property on="SP_Width" class="DigNum (strict)"("Val(Sgnl)"=w388) -> ()  [unwired: 2 in, 2 out]
        n203 = property on="SP_Height" class="DigNum (strict)"("Value"=w389) -> ()  [unwired: 2 in, 2 out]
      }
      event "SP_SetCurrentPos": Value Change {
        n204 = event-data() -> ()  [unwired: 1 in, 1 out]
        n205 = property class="VI"(reference=w405, error in=w404) -> (reference out=w406:refnum<vi>, error out=w407:errorcluster, "Front Panel.PanelBounds"=w403:T9)
        n206 = Unbundle By Name(w403) -> ("Left"=w401:i16, "Top"=w402:i16)
        n207 = property on="SP_Left" class="DigNum (strict)"("Val(Sgnl)"=w401) -> ()  [unwired: 2 in, 2 out]
        n208 = property on="SP_Top" class="DigNum (strict)"("Value"=w402) -> ()  [unwired: 2 in, 2 out]
      }
      event "SP_Scale": Value Change {
        n209 = event-data() -> ("NewVal"=w414:bool)  [unwired: 1 in]
        n210 = property class="VI"(reference=w408, error in=w418) -> (reference out=w417:refnum<vi>, error out=w416:errorcluster, "Panel"=w409:refnum<vi>)
        n211 = Select(t=T3."Scale All Objects" ("Scaling Mode"), s=w414, f=T3."No Scaling" ("Scaling Mode")) -> (s? t:f=w411:T3)
        n212 = property class="Pnl"(reference=w409) -> ("Panes[]"=w415:refnum<vi>[])  [unwired: 1 in, 2 out]
        n213 = Index Array(array=w415) -> (element=w410:refnum<vi>)  [unwired: 1 in]
        n214 = invoke class="Pane" method="Set Scaling"(reference=w410, "ScalingMode"=w411) -> ()  [unwired: 3 in, 5 out]
      }
      event "Window behavior", "Hide when LabVIEW in not active": Value Change {
        n215 = event-data() -> ()  [unwired: 1 in, 6 out]
        n216 = case shown="\"Default\"" "Window behavior" {
          tunnel: [T7."Default" ("Front Panel Window:Behavior") w430 T7."Modal" ("Front Panel Window:Behavior")] -> w421
          tunnel: "Hide when LabVIEW in not active" -> [_ w433 _]
          tunnel: [T4."Disabled and Grayed Out" ("Disabled") T4."Enabled" ("Disabled") T4."Disabled and Grayed Out" ("Disabled")] -> w419
          frame "Default" {
          }
          frame "Floating" {
            n217 = Select(t=T7."Floating/Auto-Hide" ("Front Panel Window:Behavior"), s=w433, f=T7."Floating" ("Front Panel Window:Behavior")) -> (s? t:f=w430:T7)
          }
          frame "Modal" {
          }
        }
        n218 = property class="VI"(reference=w424, error in=w426, "FP.Behavior"=w421) -> (reference out=w423:refnum<vi>, error out=w425:errorcluster)
        n219 = property on="Hide when LabVIEW in not active" class="Bool (strict)"("DisabledEnum"=w419) -> ()  [unwired: 2 in, 2 out]
      }
      event "ToSP": Value Change {
        n220 = event-data() -> ()  [unwired: 1 in, 1 out]
        n221 = Not(x="ToSP") -> (.not. x?=w440:bool)
        n222 = Select(t=enum32{"Appearance", "Size and Position"}."Size and Position" ("Tab Control"), s="ToSP", f=enum32{"Appearance", "Size and Position"}."Appearance" ("Tab Control")) -> (s? t:f=w436:enum32{"Appearance", "Size and Position"})
        n223 = local write "ToAP"(w440) -> ()
        n224 = property on="Tab Control" class="TabCtl (strict)"(error in=w442, "Value"=w436) -> (error out=w441:errorcluster)  [unwired: 1 in, 1 out]
      }
      event "ToAP": Value Change {
        n225 = event-data() -> ()  [unwired: 1 in, 1 out]
        n226 = Not(x="ToAP") -> (.not. x?=w448:bool)
        n227 = Select(t=enum32{"Appearance", "Size and Position"}."Appearance" ("Tab Control"), s="ToAP", f=enum32{"Appearance", "Size and Position"}."Size and Position" ("Tab Control")) -> (s? t:f=w446:enum32{"Appearance", "Size and Position"})
        n228 = local write "ToSP"(w448) -> ()
        n229 = property on="Tab Control" class="TabCtl (strict)"(error in=w450, "Value"=w446) -> (error out=w449:errorcluster)  [unwired: 1 in, 1 out]
      }
    }
    n230 = invoke class="VI" method="Save.Instrument"(reference=w10, error in=w14) -> (reference out=w9:refnum<vi>, error out=w11:errorcluster)  [unwired: 4 in, 4 out]
    n231 = call <vilib>:"Clear Errors.vi"("error in (no error)"=w11) -> ("error out"=w12:errorcluster)  [unwired: 5 in, 1 out]
  }
